vi "Pulse Attribute, Find Transitions.vi"(6 "hysteresis (10%)":dbl=10.0 min=-100.0 max=100.0 step=1.0 format="%.1f", 7 "transitions/per pulse (4)":i32=4, 8 "error in":errorcluster, 9 "Recvy Amp (V)":dbl=-4.848716193577154 format="%.4f", 10 "Stim Amp (V)":dbl=5.126497538859063 format="%.4f", 11 "waveform":waveform(dbl)={"t0"=timestamp(3473168073.631 s since 1904-01-01), "dt"=1e-08, "Y"=[], "attributes"=variant("Average Size"=variant(dbl 15.0), "NSamp"=variant(dbl 400000.0), "Resistance (ohms)"=variant(dbl 500.0), "Samp Freq (MHz)"=variant(dbl 100.0), "dt (us)"=variant(dbl 0.01))}) -> (0 "error out":errorcluster, 2 "transitions":dbl[][](array[numeric]), 3 "waveform dup":waveform(dbl)={"t0"=timestamp(3473168166.8500004 s since 1904-01-01), "dt"=nan, "Y"=[], "attributes"=variant("Average Size"=variant(dbl 15.0), "NSamp"=variant(dbl 113636.0), "Resistance (ohms)"=variant(dbl 10000.0), "Samp Freq (MHz)"=variant(dbl 0.5), "dt (us)"=variant(dbl 2.0))})   [LabVIEW 2010]
uses:
  <vilib>/measure/mamon.llb/Trigger Detection for 1 Channel.vi
  <vilib>/measure/NI_MAPro.lvlib
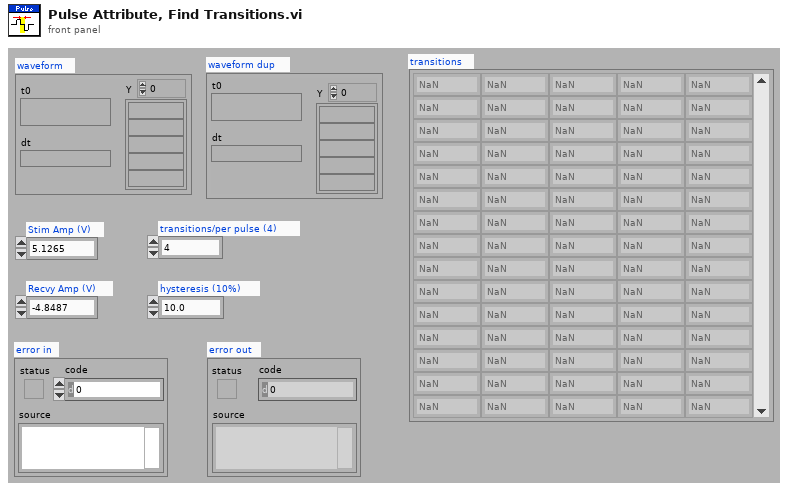
[diagram p1: front panel]
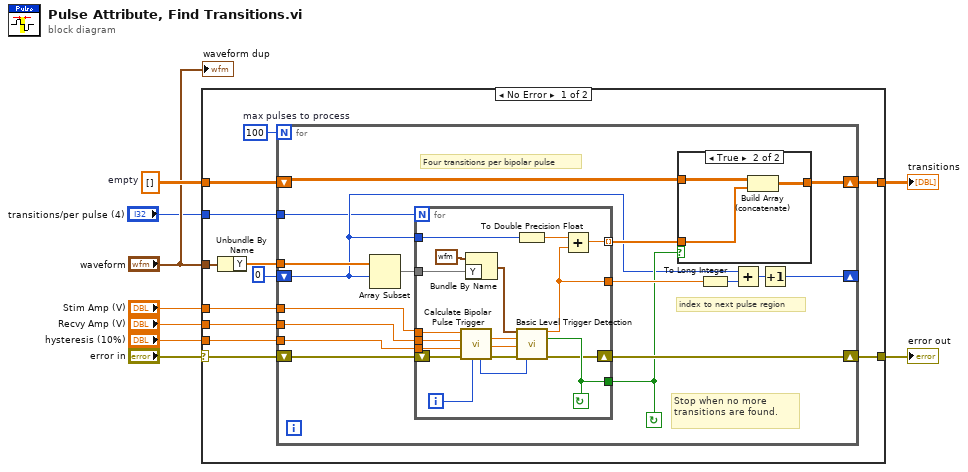
[diagram p0: block diagram]
diagram:
  w6 = dbl[][] []  # empty
  n1 = case shown="No Error" "error in" {
    selector: "error in" -> [w16 w62]
    tunnel: "Recvy Amp (V)" -> [w21 _]
    tunnel: [w20 w62] -> w8
    tunnel: "Stim Amp (V)" -> [w19 _]
    tunnel: w6 -> [w12 w61]
    tunnel: [w11 w61] -> w2
    tunnel: "waveform" -> [w14 _]
    tunnel: "hysteresis (10%)" -> [w13 _]
    tunnel: "transitions/per pulse (4)" -> [w10 _]
    frame No Error {
      w17 = 100  # max pulses to process
      n2 = Unbundle By Name(w14) -> ("Y"=w15:dbl[])
      n3 = for {
        N: w17 -> [_]
        tunnel: w21 -> [w38]
        tunnel: w19 -> [w36]
        shift-right: [w28] -> _
        shift-left: 0 ("Max Transitions") -> [w23]
        shift-right: [w31] -> w11
        shift-left: w12 -> [w32]
        shift-right: [w37] -> w20
        shift-left: w16 -> [w35]
        tunnel: w15 -> [w25]
        tunnel: w13 -> [w24]
        tunnel: w10 -> [w22]
        stop <- w26 continue-if-true
        # "index to next pulse region"
        # "Stop when no more transitions are found."
        # "Four transitions per bipolar pulse"
        n4 = Array Subset(array=w25, index=w23) -> (w34:dbl[])  [unwired: 1 in]
        n5 = for {
          N: w22 -> [_]
          shift-right: [w52] -> w37
          shift-left: w35 -> [w57]
          tunnel: w38 -> [w56]
          tunnel: w36 -> [w55]
          tunnel: [w53] -> w26
          tunnel: [w45] -> w27 mode=indexing
          tunnel: w34 -> [w49]
          tunnel: [w46] -> w33
          tunnel: w24 -> [w47]
          tunnel: w23 -> [w44]
          i -> [w58]
          stop <- w53 continue-if-true
          n6 = call "Calculate Bipolar Pulse Trigger.vi"("pulse index"=w58, "error in"=w57, "hysteresis (10%)"=w47, "Recvy Amp (V)"=w56, "Stim Amp (V)"=w55) -> ("error out"=w54:errorcluster, "hysteresis (V)"=w48:dbl, "trigger level (V)"=w59:dbl, "trigger slope"=w60:u16)  [unwired: 3 in]
          n7 = Bundle By Name(cluster=waveform(dbl) {"t0"=timestamp(0 s since 1904-01-01), "dt"=1.0, "Y"=[]} ("waveform"), "Y"=w49) -> (w50:waveform(dbl))
          n8 = To Double Precision Float(number=w44) -> (double precision float=w43:dbl)
          n9 = call-poly <vilib>:"Basic Level Trigger Detection.vi"("signal in"=w50, "level"=w59, "hysteresis"=w48, "error in (no error)"=w54, "trigger slope"=w60) -> ("trigger location"=w46:dbl, "trigger detected?"=w53:bool, "error out"=w52:errorcluster)  [unwired: 8 in]
          n10 = Add(x=w43, y=w46) -> (x+y=w45:dbl)
        }
        n11 = case shown="True" w26 {
          tunnel: w32 -> [w39 w42]
          tunnel: [w39 w41] -> w31
          tunnel: w27 -> [_ w40]
          frame False {
          }
          frame True {
            n12 = Build Array (concatenate)(w42, w40) -> (w41:dbl[][])
          }
        }
        n13 = To Long Integer(number=w33) -> (32bit integer=w30:i32)
        n14 = Add(x=w23, y=w30) -> (x+y=w29:i32)
        n15 = Increment(x=w29) -> (x+1=w28:i32)
      }
    }
    frame Error {
    }
  }
  "error out" <- w8
  "transitions" <- w2
  "waveform dup" <- "waveform"
